vi "ProcessName.vi"() -> (1 "process name":string)   [LabVIEW 2017, in "McsaFpgaBitfileManager.lvlib"]
uses:
  <vilib>/addons/InsightCM/Devices/Shared/Mcsa/McsaFpgaBitfileManager/McsaFpgaBitfileManager.lvlib
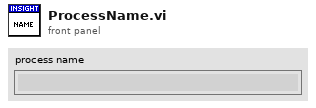
[diagram p1: front panel]
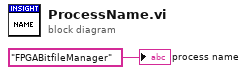
[diagram p0: block diagram]
diagram:
  "process name" <- "FPGABitfileManager" ("ProcessName")
